vi "DLPCA-200-SubVI.vi"() -> ()   [LabVIEW 2025]
uses:
  <userlib>/_FEMTO Messtechnik GmbH/LUCI-10/_TypeDefs/Choose_Device_Enum.ctl
  <userlib>/_FEMTO Messtechnik GmbH/LUCI-10/Control/Set_Gain_DLPCA-200.vi
  <userlib>/_FEMTO Messtechnik GmbH/LUCI-10/FEMTO_LUCI-10.lvlib
panel:
  in  "Femto Gain V/A":dbl(ring) items=["1E3"=1.0, "1E4"=2.0, "1E5"=3.0, "1E6"=4.0, "1E7"=5.0, "1E8"=6.0, "1E9"=7.0]
  out "Numeric":dbl
  in  "Available LUCI-10 Devices":i32(listbox)
  in  "Info":bool
  out "Overload":bool
  in  "Rahmen":bool
  in  "stop":bool
  out "LED":bool
  in  "Check LUCI":bool
  out "String_Product":string
  in  "Product_String":bool
  # "Remote Control LUCI-10 DLPCA-200"
  # "DLPCA-200"
  # "Configuration"
  # "Gain Setting"
  # "5"
  # "6"
  # "7"
  # "8"
  # "9"
  # "10"
  # "11"
  # "10"
  # "10"
  # "10"
  # "10"
  # "10"
  # "10"
  # "10"
  # "H"
  # "V/A"
  # "Device Information"
  # "L"
  # "3"
  # "4"
  # "5"
  # "6"
  # "7"
  # "8"
  # "9"
  # "10"
  # "10"
  # "10"
  # "10"
  # "10"
  # "10"
  # "10"
  # "500"
  # "500"
  # "400"
  # "200"
  # "50"
  # "7"
  # "1"
  # "kHz"
  # "Overload"
  # "Coupling"
  # "AC"
  # "DC"
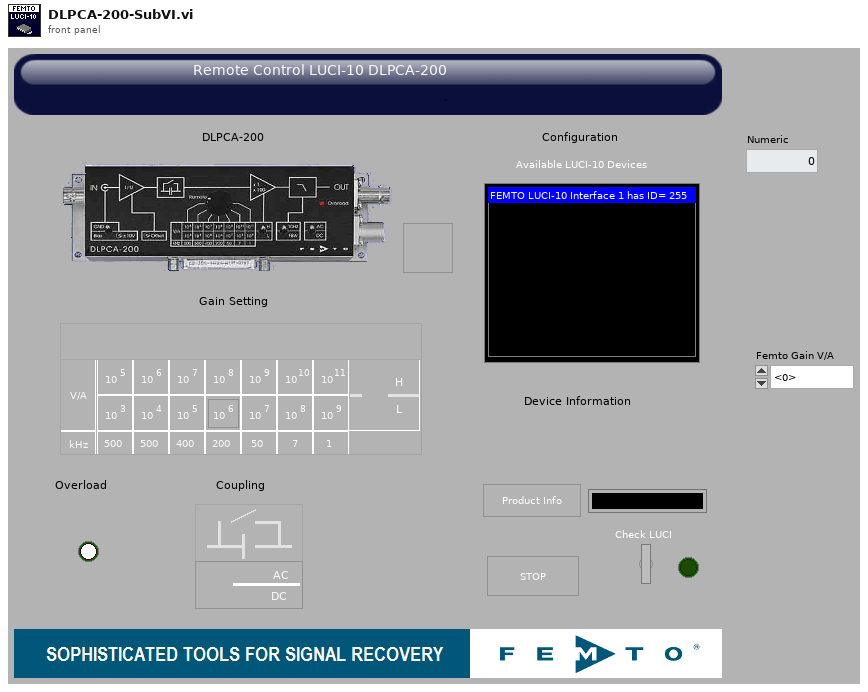
[diagram p1: front panel]
types:
  T1 = typedef "FEMTO_LUCI-10.lvlib/Choose_Device_Enum.ctl" = enum16{"DDPCA-300", "DLPCA-200", "DHPCA-100", "OE-200", "OE-300", "LIA-MV-150-S", "LIA-MV-150-D", "LIA-MV-200-L", "LIA-MV-200-H", "LIA-MVD-200-L", "LIA-MVD-200-H", "DLPVA-100-BUN-S", "DLPVA-100-BLN-S", "DLPVA-100-B-S", "DLPVA-100-B-D", "DLPVA-100-F-S", "DLPVA-100-F-D", "DHPVA-100", "DHPVA-200", "DUPVA-1-60", "DUPVA-1-70"}
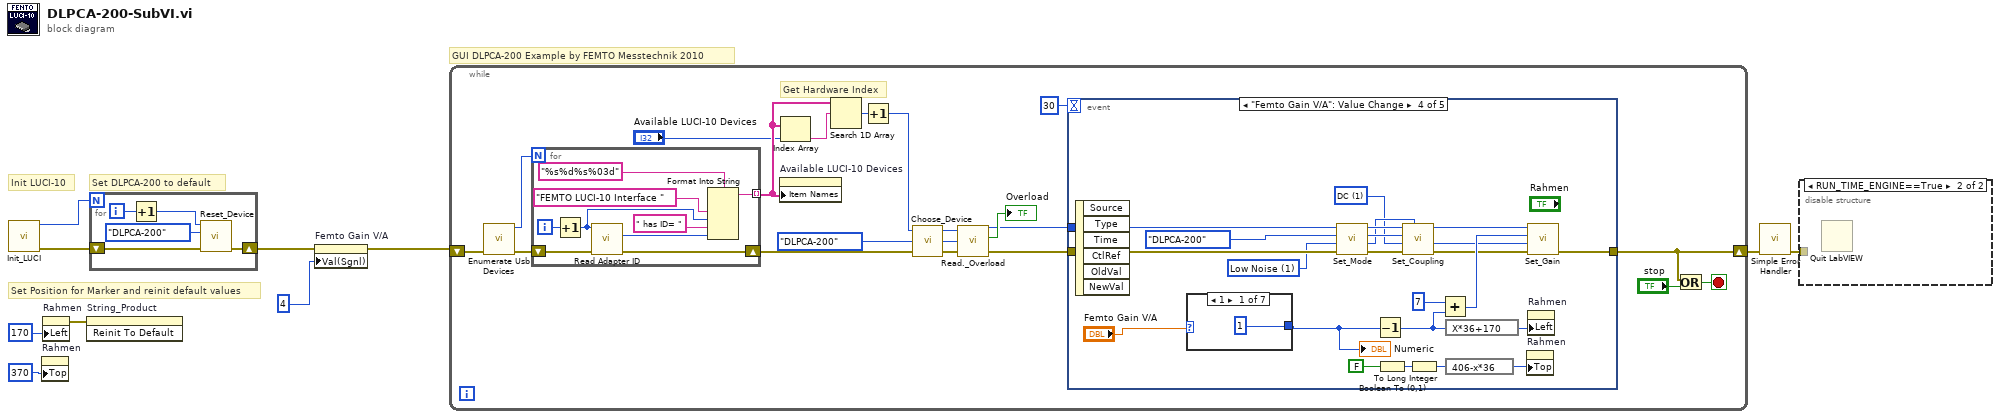
[diagram p0: block diagram]
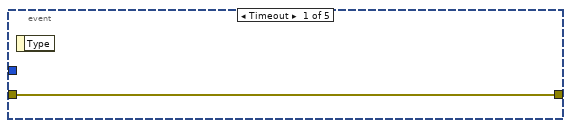
[diagram p3: hidden frame]
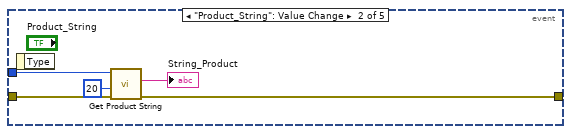
[diagram p4: hidden frame]
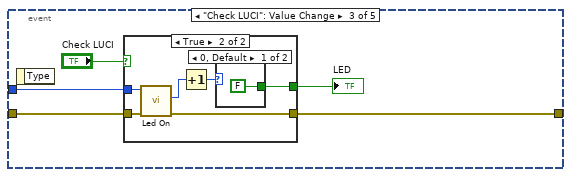
[diagram p5: hidden frame]
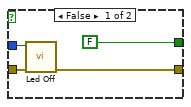
[diagram p6: hidden frame]
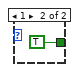
[diagram p7: hidden frame]
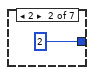
[diagram p8: hidden frame]
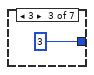
[diagram p9: hidden frame]
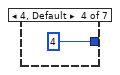
[diagram p10: hidden frame]
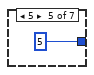
[diagram p11: hidden frame]
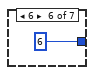
[diagram p12: hidden frame]
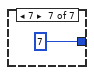
[diagram p13: hidden frame]
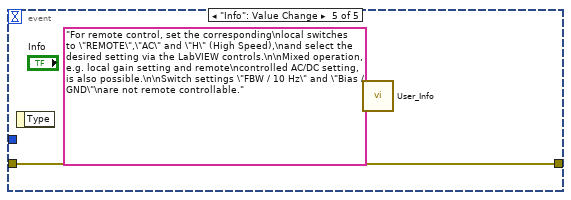
[diagram p14: hidden frame]
diagram:
  # "Set DLPCA-200 to default"
  # "Set Position for Marker and reinit default values"
  # "Init LUCI-10"
  # "GUI DLPCA-200 Example by FEMTO Messtechnik 2010"
  n1 = call <userlib>:"Init_LUCI.vi"() -> ("error out"=w7:errorcluster, "Number of Devices"=w8:i32)  [unwired: 10 in]
  n2 = property on="Rahmen" class="Bool"("Top"=370 ("Position:Top")) -> ()  [unwired: 2 in, 2 out]
  n3 = property on="Rahmen" class="Bool"("Left"=170 ("Position:Left")) -> (error out=w6:errorcluster)  [unwired: 2 in, 1 out]
  n4 = invoke on="String_Product" class="Str" method="Reinit To Default"(error in=w6) -> ()  [unwired: 2 in, 3 out]
  n5 = for {
    N: w8 -> [_]
    shift-right: [w11] -> w3
    shift-left: w7 -> [w12]
    i -> [w15]
    n6 = Increment(x=w15) -> (x+1=w13:i32)
    n7 = call <userlib>:"Reset_Device.vi"("error in (no error)"=w12, "Choose_Device"=Choose_Device_Enum."DLPCA-200", "Index"=w13) -> ("error out"=w11:errorcluster)  [unwired: 4 in, 2 out]
  }
  n8 = property on="Femto Gain V/A" class="Ring (strict)"(error in=w3, "Val(Sgnl)"=4) -> (error out=w2:errorcluster)  [unwired: 1 in, 1 out]
  n9 = while {
    shift-right: [w16] -> w5
    shift-left: w2 -> [w25]
    stop <- w17 stop-if-true
    # "Get Hardware Index"
    n10 = call <userlib>:"Enumerate Usb Devices.vi"("error in (no error)"=w25) -> ("error out"=w18:errorcluster, "function return"=w26:i32)  [unwired: 9 in]
    n11 = for {
      N: w26 -> [_]
      tunnel: [w38] -> w22 mode=indexing
      shift-right: [w37] -> w19
      shift-left: w18 -> [w36]
      i -> [w39]
      n12 = Increment(x=w39) -> (x+1=w44:i32)
      n13 = call <userlib>:"Read Adapter ID.vi"("error in (no error)"=w36, "index"=w44) -> ("error out"=w37:errorcluster, "id out"=w43:i32)  [unwired: 7 in, 1 out]
      n14 = Format Into String(format string="%s%d%s%03d", "FEMTO LUCI-10 Interface ", w44, " has ID= ", w43) -> (resulting string=w38:string)  [unwired: 2 in, 1 out]
    }
    n15 = property on="Available LUCI-10 Devices" class="LstBox (strict)"("Item Names"=w22) -> ()  [unwired: 2 in, 2 out]
    n16 = Index Array(array=w22, index="Available LUCI-10 Devices") -> (element=w23:string)
    n17 = Search 1D Array(1D array=w22, element=w23) -> (index of element=w24:i32)  [unwired: 1 in]
    n18 = Increment(x=w24) -> (x+1=w20:i32)
    n19 = call <userlib>:"Choose_Device.vi"("error in (no error)"=w19, "Choose_Device"=Choose_Device_Enum."DLPCA-200", "Index"=w20) -> ("error out"=w31:errorcluster, "Device_type"=w32:T1, "Index_Out"=w33:i32)
    n20 = call <userlib>:"Read._Overload.vi"("Index"=w33, "Choose_Device"=w32, "error in (no error)"=w31) -> ("Index_Out"=w27:i32, "Overload"=→"Overload":bool, "error out"=w28:errorcluster)  [unwired: 1 out]
    n21 = event shown="[3] \"Femto Gain V/A\": Value Change" {
      selector: _ -> [_ _ _ _ _]
      dyn-events: _ -> [_ _ _ _ _]
      timeout: 30 -> [_ _ _ _ _]
      tunnel: w28 -> [w45 w48 w53 w75 w98]
      tunnel: w27 -> [_ w50 w54 w86 _]
      tunnel: [w45 w46 w51 w73 w98] -> w16
      event Timeout {
        n22 = event-data() -> ()  [unwired: 1 in, 1 out]
      }
      event "Product_String": Value Change {
        n23 = event-data() -> ()  [unwired: 1 in, 1 out]
        n24 = call <userlib>:"Get Product String.vi"("error in (no error)"=w48, "size"=20, "index"=w50) -> ("error out"=w46:errorcluster, "string out"=→"String_Product":string)  [unwired: 6 in, 1 out]
      }
      event "Check LUCI": Value Change {
        n25 = event-data() -> ()  [unwired: 1 in, 1 out]
        n26 = case shown="True" "Check LUCI" {
          tunnel: w54 -> [w59 w65]
          tunnel: w53 -> [w58 w64]
          tunnel: [FALSE w61] -> w52
          tunnel: [w56 w60] -> w51
          frame False {
            n27 = call <userlib>:"Led Off.vi"("error in (no error)"=w58, "index"=w59) -> ("error out"=w56:errorcluster)  [unwired: 8 in, 1 out]
          }
          frame True {
            n28 = call <userlib>:"Led On.vi"("error in (no error)"=w64, "index"=w65) -> ("error out"=w60:errorcluster, "function_return"=w63:i32)  [unwired: 7 in, 1 out]
            n29 = Increment(x=w63) -> (x+1=w62:i32)
            n30 = case shown="0, Default" w62 {
              tunnel: [FALSE TRUE] -> w61
              frame 0, Default {
              }
              frame 1 {
              }
            }
          }
        }
        "LED" <- w52
      }
      event "Femto Gain V/A": Value Change {
        w72 = u16 1 items=["AC", "DC"] ("Set Coupling")
        w70 = u16 1 items=["High Speed", "Low Noise"] ("Set Mode")
        n31 = event-data() -> ()  [unwired: 1 in, 6 out]
        n32 = case shown="1" "Femto Gain V/A" {
          tunnel: [1 2 3 4 5 6 7] -> w69
          frame 1 {
          }
          frame 2 {
          }
          frame 3 {
          }
          frame 4, Default {
          }
          frame 5 {
          }
          frame 6 {
          }
          frame 7 {
          }
        }
        "Numeric" <- w69
        n33 = call <userlib>:"Set_Mode.vi"("error in (no error)"=w75, "Set Mode"=w70, "Choose_Device"=Choose_Device_Enum."DLPCA-200", "Index"=w86) -> ("error out"=w80:errorcluster, "Status_out"=w81:i32, "Device_type"=w82:T1, "Index_Out"=w83:i32)  [unwired: 1 in]
        n34 = Decrement(x=w69) -> (x-1=w84:i32)
        n35 = Boolean To (0,1)(Boolean=FALSE) -> (0, 1=w90:i16)
        n36 = call <userlib>:"Set_Coupling.vi"("Status"=w81, "error in (no error)"=w80, "Set Coupling"=w72, "Choose_Device"=w82, "Index"=w83) -> ("error out"=w76:errorcluster, "Status_out"=w77:i32, "Index_Out"=w79:i32)  [unwired: 1 out]
        n37 = To Long Integer(number=w90) -> (32bit integer=w89:i32)
        n38 = Add(x=7, y=w84) -> (x+y=w78:i32)
        n39 = expression code="X*36+170"(w84) -> (w88:i32)
        n40 = expression code="406-x*36"(w89) -> (w87:i32)
        n41 = property on="Rahmen" class="Bool"("Top"=w87) -> ()  [unwired: 2 in, 2 out]
        n42 = call-poly <userlib>:"Set_Gain.vi"("error in"=w76, "Status"=w77, "Gain  [V/A]"=w78, "index"=w79) -> ("error out"=w73:errorcluster)  [unwired: 2 out]
        n43 = property on="Rahmen" class="Bool"("Left"=w88) -> ()  [unwired: 2 in, 2 out]
      }
      event "Info": Value Change {
        n44 = event-data() -> ()  [unwired: 1 in, 1 out]
        n45 = call <userlib>:"User_Info.vi"("String"="For remote control, set the corresponding\nlocal switches to \"REMOTE\",\"AC\" and \"H\" (High Speed),\nand select the desired setting via the LabVIEW controls.\n\nMixed operation, e.g. local gain setting and remote\ncontrolled AC/DC setting, is also possible.\n\nSwitch settings \"FBW / 10 Hz\" and \"Bias / GND\"\nare not remote controllable.") -> ()  [unwired: 1 in]
      }
    }
    n46 = Or(x=w16, y="stop") -> (x .or. y?=w17:bool)
  }
  n47 = call <vilib>:"Simple Error Handler.vi"("error in (no error)"=w5) -> ("error out"=w4:errorcluster)  [unwired: 4 in, 4 out]
  n48 = disable-structure shown="RUN_TIME_ENGINE==True" {
    disable-tunnel: w4 -> [_ _]
    frame condition #0 (active) {
    }
    frame condition #1 {
      n49 = Quit LabVIEW() -> ()  [unwired: 1 in]
    }
  }
